vi "set_serial.vi"(6 "timeout (25000ms)":i32=25000, 8 "error in (no error)":errorcluster, 10 "Serial number":string, 11 "daemon reference in":refnum<k5>) -> (0 "error out":errorcluster, 2 "response":string, 3 "daemon reference out":refnum<k5>, 5 "command out":string="random")   [LabVIEW 2017]
doc: "<b>Command: </b>\"set_ddm_sn\"\n\n<b>Description: </b> This command set ddm serial number.\n\n<b>Parameters: </b> Serial number\n____________________________________________\nDIPC 692 Daemon API 10.0.0.1\nSam Tee - Dyson Technology Ltd\nCopyright (c) 2024, Dyson Technology Ltd"
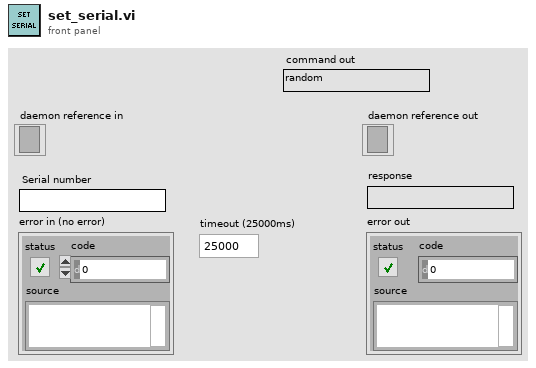
[diagram p1: front panel]
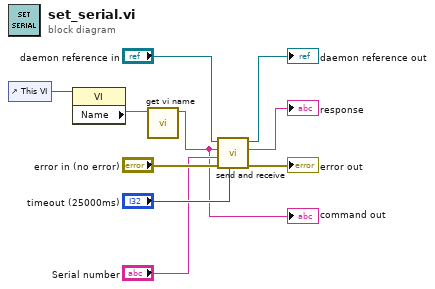
[diagram p0: block diagram]
diagram:
  n1 = control-ref of="This VI"() -> (w4:refnum<vi>)
  n2 = property class="VI"(reference=w4) -> ("Name"=w2:string)  [unwired: 1 in, 2 out]
  n3 = call "get vi name.vi"("library.lvlib:name.vi"=w2) -> ("vi name"=w1:string)  [unwired: 10 in]
  "command out" <- w1
  n4 = call "send and receive.vi"("timeout (25000ms)"="timeout (25000ms)", "error in (no error)"="error in (no error)", "data"="Serial number", "command"=w1, "daemon reference in"="daemon reference in") -> ("error out"=→"error out":errorcluster, "response"=→"response":string, "daemon reference out"=→"daemon reference out":refnum<k5>)  [unwired: 4 in]
